vi "Main.vi"() -> ()   [LabVIEW 2019]
doc: "Simple string based state machine."
uses:
  <vilib>/Utility/error.llb/Error Cluster From Error Code.vi
  <vilib>/ErrorRing/Error Ring.xnode
  Support VIs/Communication/Queues/MHL/MHL.lvlib
  Support VIs/Modules/Deep Thought/Deep Thought.lvlib
  Support VIs/Communication/Notifiers/Sequencer/Sequencer Handshake.lvlib
panel:
  out "Deep Thought":string
  in  "Ultimate Question":bool
  in  "Ultimate Answer":bool
  in  "Stop":bool
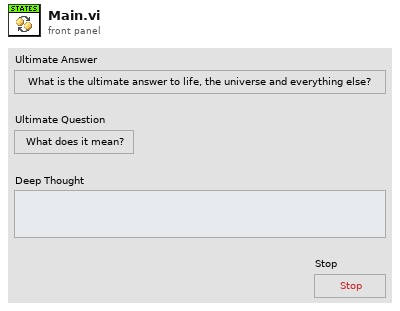
[diagram p1: front panel]
types:
  T1 = typedef "Events.ctl" = cluster{"Stop":refnum<user-event>}
  T2 = enum16{"Create Event", "Generate Event", "Destroy Event"}
  T3 = enum16{"Obtain", "Enqueue", "Get Queue", "Flush", "Release"}
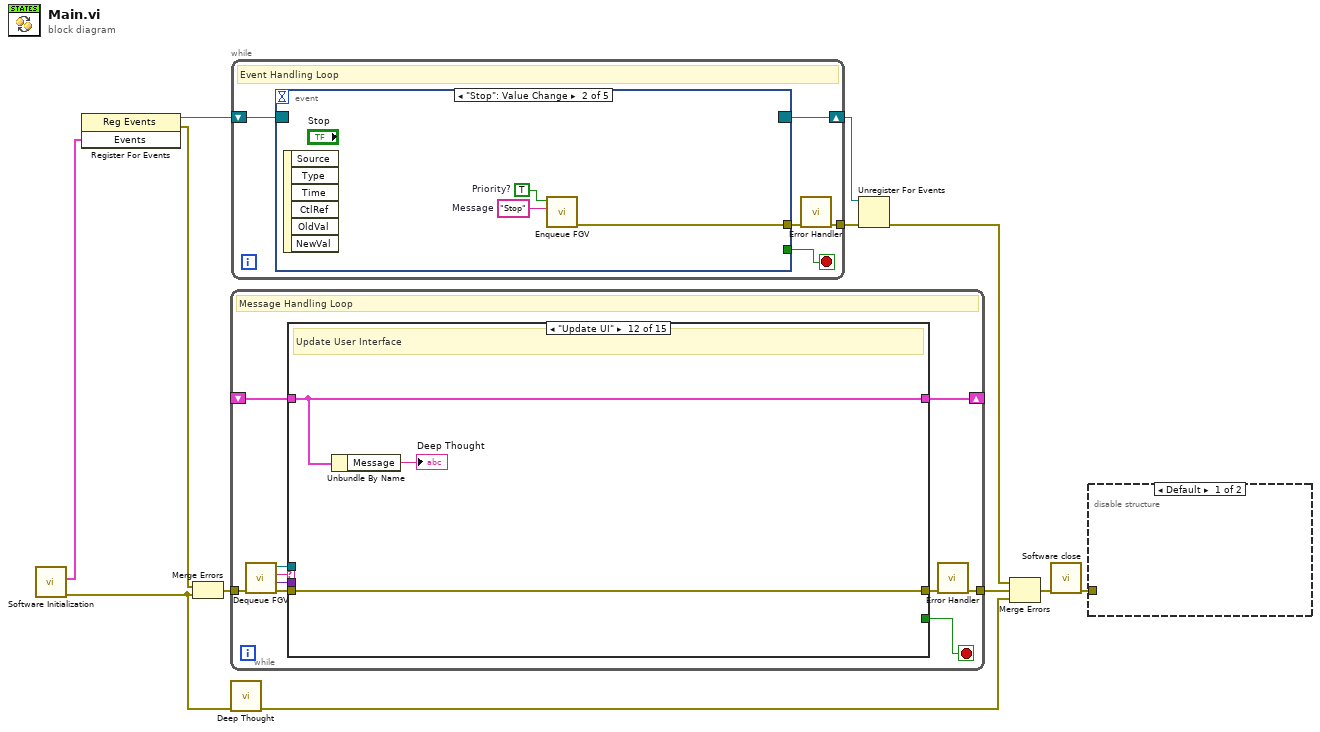
[diagram p0: block diagram]
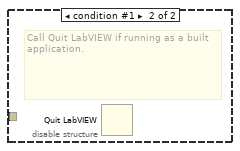
[diagram p2: hidden frame]
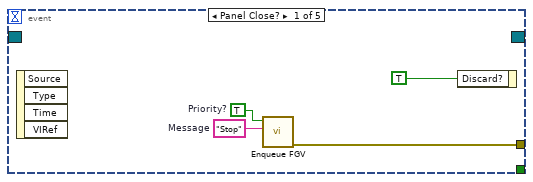
[diagram p3: hidden frame]
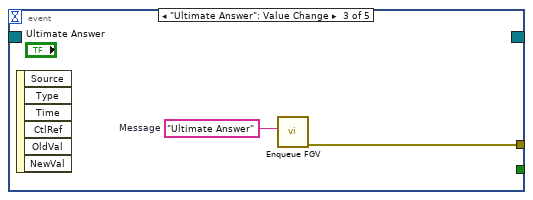
[diagram p4: hidden frame]
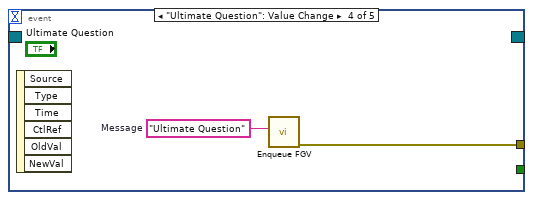
[diagram p5: hidden frame]
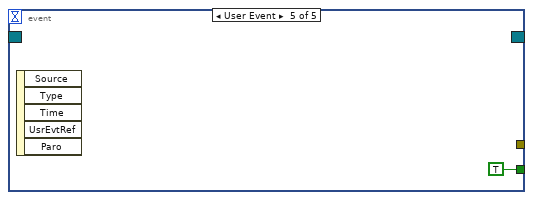
[diagram p6: hidden frame]
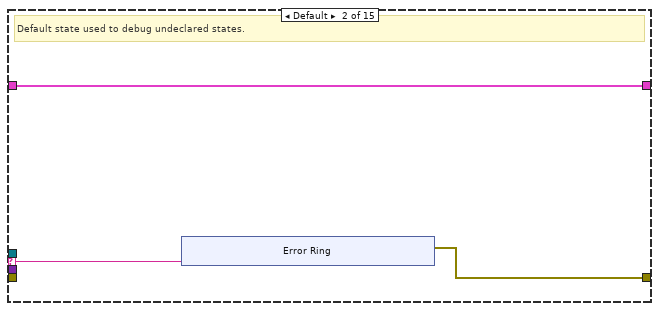
[diagram p8: hidden frame]
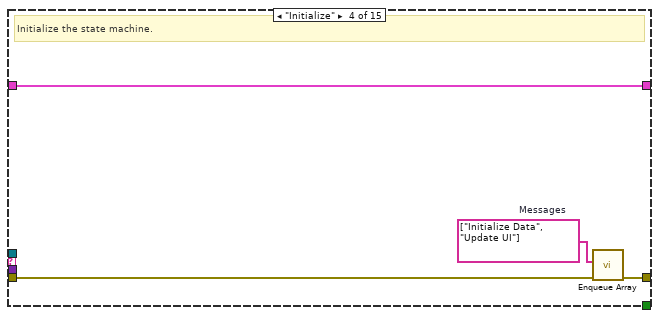
[diagram p10: hidden frame]
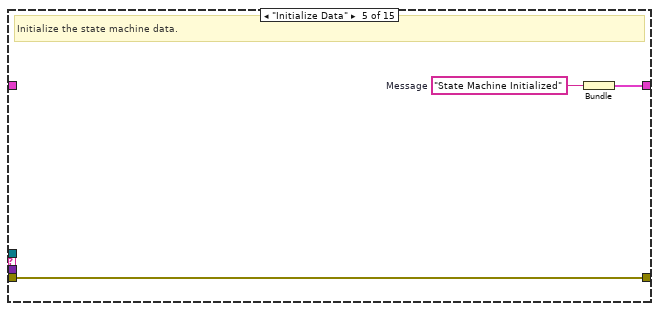
[diagram p11: hidden frame]
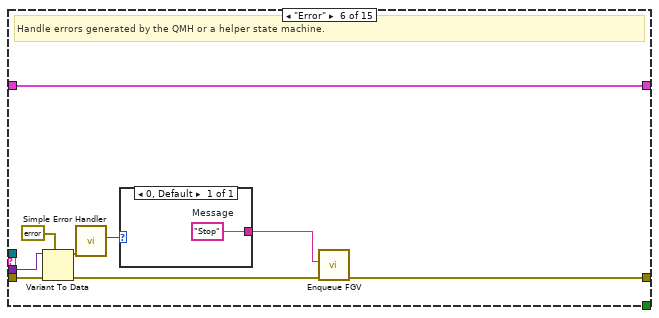
[diagram p12: hidden frame]
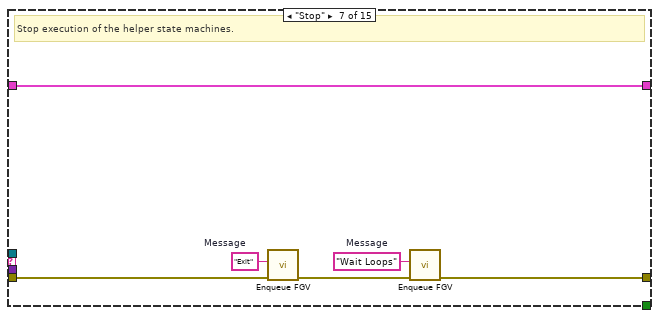
[diagram p13: hidden frame]
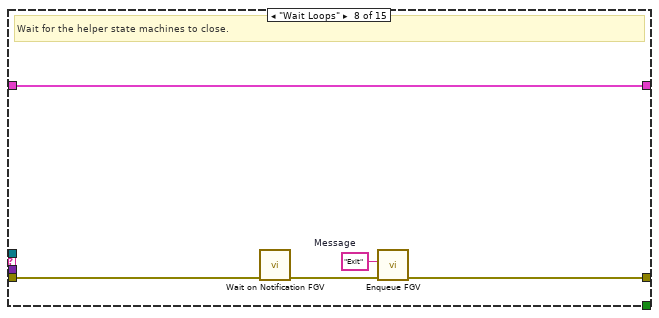
[diagram p14: hidden frame]
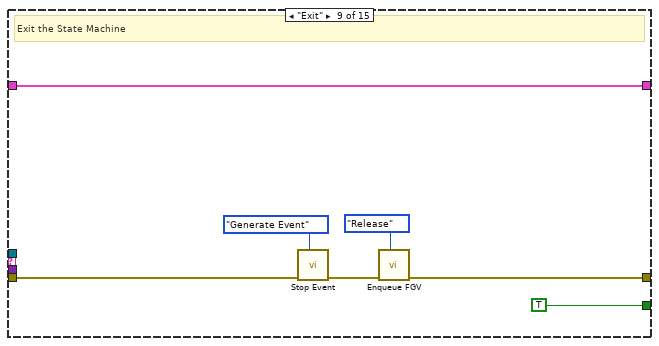
[diagram p15: hidden frame]
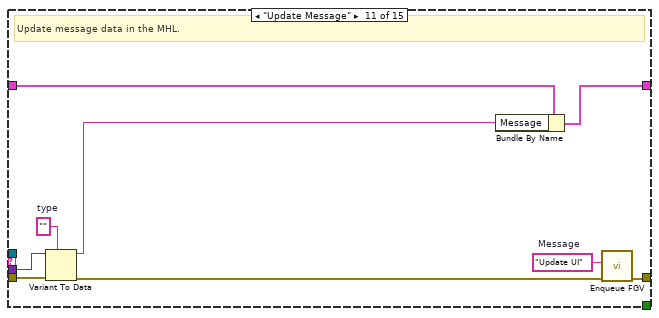
[diagram p17: hidden frame]
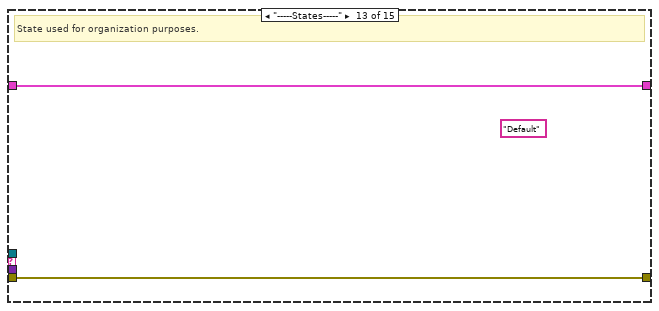
[diagram p18: hidden frame]
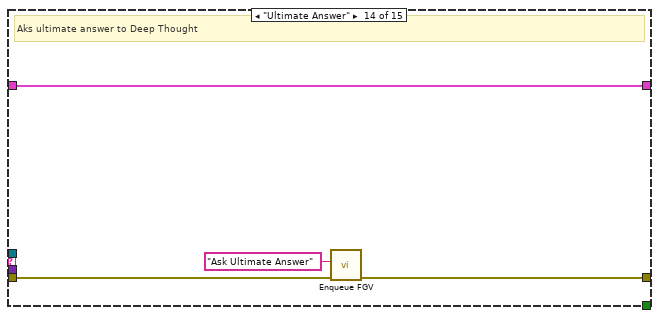
[diagram p19: hidden frame]
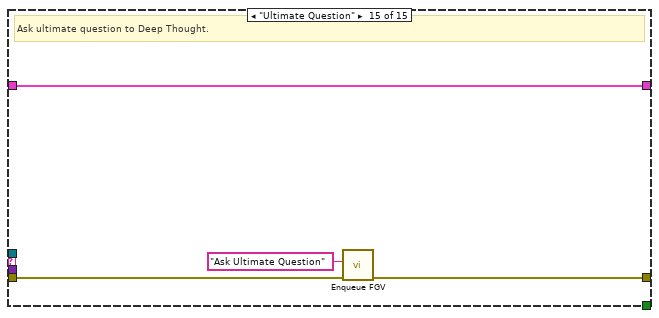
[diagram p20: hidden frame]
diagram:
  n1 = call "Software Initialization.vi"() -> ("error out"=w2:errorcluster, "Events"=w10:T1)  [unwired: 10 in]
  n2 = register-events(w10) -> (reference out=w11:refnum<event-registration>, error out=w8:errorcluster)  [unwired: 2 in]
  n3 = Merge Errors(w8, w2) -> (w9:errorcluster)
  n4 = while {
    shift-right: [w21] -> _
    shift-left: _ -> [w22]
    tunnel: w9 -> [w20]
    tunnel: [w18] -> w5
    stop <- w13 stop-if-true
    # "Message Handling Loop"
    n5 = call "Dequeue FGV.vi"("error in"=w20) -> ("error out"=w19:errorcluster, "Message Data"=w15:variant, "Message"=w16:string, "queue out"=w14:refnum<queue>)  [unwired: 7 in]
    n6 = case shown="\"Update UI\"" w16 {
      selector: w16 -> [_ w26 _ _ _ _ _ _ _ _ _ _ _ _ _]
      tunnel: w19 -> [w24 _ w36 w39 w41 w51 w56 w63 w66 w73 w80 w83 w87 w91 w95]
      tunnel: [w24 w25 w36 w40 w41 w46 w58 w61 w69 w73 w76 w83 w87 w90 w94] -> w17
      tunnel: [_ _ _ _ _ _ _ _ TRUE _ _ _ _ _ _] -> w13
      tunnel: w22 -> [w23 w27 w35 w37 _ w52 w59 w64 w70 w72 w82 w85 w86 w88 w92]
      tunnel: [w23 w27 w35 w37 w42 w52 w59 w64 w70 w72 w81 w85 w86 w88 w92] -> w21
      tunnel: w15 -> [_ _ _ _ _ w50 _ _ _ _ w79 _ _ _ _]
      tunnel: w14 -> [_ _ _ _ _ _ _ _ _ _ _ _ _ _ _]
      frame "-----Debug-----" {
        # "State used for organization purposes."
      }
      frame Default {
        # "Default state used to debug undeclared states."
        n7 = xnode "Error Ring"("parameter 0"=w26) -> ("error out"=w25:errorcluster)
      }
      frame "-----Core-----" {
        # "State used for organization purposes."
      }
      frame "Initialize" {
        w38 = string[] ["Initialize Data", "Update UI"]  # Messages
        # "Initialize the state machine."
        n8 = call "Enqueue Array.vi"("error in"=w39, "Messages"=w38) -> ("error out"=w40:errorcluster)  [unwired: 9 in]
      }
      frame "Initialize Data" {
        w43 = "State Machine Initialized"  # Message
        # "Initialize the state machine data."
        n9 = Bundle("Message"=w43) -> (w42:cluster{"Message":string})  [unwired: 1 in]
      }
      frame "Error" {
        # "Handle errors generated by the QMH or a helper state machine."
        n10 = Variant To Data(error in=w51, type=errorcluster {"status"=FALSE, "code"=0, "source"=""} ("error constant"), Variant=w50) -> (data=w48:errorcluster, error out=w47:errorcluster)
        n11 = call <vilib>:"Simple Error Handler.vi"("error in (no error)"=w48) -> ("code out"=w45:i32)  [unwired: 4 in, 4 out]
        n12 = case shown="0, Default" w45 {
          tunnel: [w53] -> w44
          frame 0, Default {
            w53 = "Stop"  # Message
          }
        }
        n13 = call "Enqueue FGV.vi"("error in"=w47, "Message"=w44) -> ("error out"=w46:errorcluster)  [unwired: 8 in, 1 out]
      }
      frame "Stop" {
        w54 = "Wait Loops"  # Message
        w55 = "Exit"  # Message
        # "Stop execution of the helper state machines."
        n14 = call "Enqueue FGV.vi"("error in"=w56, "Message"=w55) -> ("error out"=w57:errorcluster)  [unwired: 8 in, 1 out]
        n15 = call "Enqueue FGV.vi"("error in"=w57, "Message"=w54) -> ("error out"=w58:errorcluster)  [unwired: 8 in, 1 out]
      }
      frame "Wait Loops" {
        w60 = "Exit"  # Message
        # "Wait for the helper state machines to close."
        n16 = call "Wait on Notification FGV.vi"("error in"=w63) -> ("error out"=w62:errorcluster)  [unwired: 8 in, 2 out]
        n17 = call "Enqueue FGV.vi"("error in"=w62, "Message"=w60) -> ("error out"=w61:errorcluster)  [unwired: 8 in, 1 out]
      }
      frame "Exit" {
        # "Exit the State Machine"
        n18 = call "Stop Event.vi"("Actions"=T2."Generate Event", "error in"=w66) -> ("error out"=w65:errorcluster)  [unwired: 8 in, 1 out]
        n19 = call "Enqueue FGV.vi"("Actions"=T3."Release", "error in"=w65) -> ("error out"=w69:errorcluster)  [unwired: 8 in, 1 out]
      }
      frame "-----User Interface-----" {
        # "State used for organization purposes."
      }
      frame "Update Message" {
        w74 = "Update UI"  # Message
        w78 = ""  # type
        # "Update message data in the MHL."
        n20 = Variant To Data(error in=w80, type=w78, Variant=w79) -> (data=w77:string, error out=w75:errorcluster)
        n21 = Bundle By Name(cluster=w82, "Message"=w77) -> (w81:cluster{"Message":string})
        n22 = call "Enqueue FGV.vi"("error in"=w75, "Message"=w74) -> ("error out"=w76:errorcluster)  [unwired: 8 in, 1 out]
      }
      frame "Update UI" {
        # "Update User Interface"
        n23 = Unbundle By Name(w85) -> ("Message"=→"Deep Thought":string)
      }
      frame "-----States-----" {
        (unwired) "Default" ("State")
        # "State used for organization purposes."
      }
      frame "Ultimate Answer" {
        # "Aks ultimate answer to Deep Thought"
        n24 = call "Enqueue FGV.vi"("error in"=w91, "Message"="Ask Ultimate Answer") -> ("error out"=w90:errorcluster)  [unwired: 8 in, 1 out]
      }
      frame "Ultimate Question" {
        # "Ask ultimate question to Deep Thought."
        n25 = call "Enqueue FGV.vi"("error in"=w95, "Message"="Ask Ultimate Question") -> ("error out"=w94:errorcluster)  [unwired: 8 in, 1 out]
      }
    }
    n26 = call "Error Handler.vi"("error in"=w17) -> ("dup error in"=w18:errorcluster)  [unwired: 9 in, 1 out]
  }
  n27 = call "Deep Thought.vi"("Error In"=w2) -> ("Error Out"=w1:errorcluster)  [unwired: 10 in]
  n28 = while {
    shift-right: [w97] -> w6
    shift-left: w11 -> [w100]
    tunnel: [w98] -> w7
    stop <- w96 stop-if-true
    # "Event Handling Loop"
    n29 = event shown="[1] \"Stop\": Value Change" {
      selector: w100 -> [_ _ _ _ _]
      dyn-events: [_ _ _ _ _] -> w97
      timeout: _ -> [_ _ _ _ _]
      tunnel: [w103 w105 w108 w110 _] -> w99
      tunnel: [_ _ _ _ TRUE] -> w96
      event Panel Close? {
        w101 = "Stop"  # Message
        w102 = TRUE  # Priority?
        # "Panel Close event."
        n30 = event-data() -> ()  [unwired: 1 in, 4 out]
        n31 = call "Enqueue FGV.vi"("Message"=w101, "Priority?"=w102) -> ("error out"=w103:errorcluster)  [unwired: 8 in, 1 out]
        n32 = event-data("Discard?"=TRUE) -> ()  [unwired: 1 in, 1 out]
      }
      event "Stop": Value Change {
        w106 = "Stop"  # Message
        w107 = TRUE  # Priority?
        # "Stop button value change event."
        n33 = event-data() -> ()  [unwired: 1 in, 6 out]
        n34 = call "Enqueue FGV.vi"("Message"=w106, "Priority?"=w107) -> ("error out"=w105:errorcluster)  [unwired: 8 in, 1 out]
      }
      event "Ultimate Answer": Value Change {
        w109 = "Ultimate Answer"  # Message
        # "Ultimate Answer button value change event."
        n35 = event-data() -> ()  [unwired: 1 in, 6 out]
        n36 = call "Enqueue FGV.vi"("Message"=w109) -> ("error out"=w108:errorcluster)  [unwired: 9 in, 1 out]
      }
      event "Ultimate Question": Value Change {
        w111 = "Ultimate Question"  # Message
        # "Ultimate Question button value change event."
        n37 = event-data() -> ()  [unwired: 1 in, 6 out]
        n38 = call "Enqueue FGV.vi"("Message"=w111) -> ("error out"=w110:errorcluster)  [unwired: 9 in, 1 out]
      }
      event User Event {
        n39 = event-data() -> ()  [unwired: 1 in, 5 out]
      }
    }
    n40 = call "Error Handler.vi"("error in"=w99) -> ("dup error in"=w98:errorcluster)  [unwired: 9 in, 1 out]
  }
  n41 = Unregister For Events(event registration refnum=w6, error in=w7) -> (error out=w4:errorcluster)
  n42 = Merge Errors(w4, w5, w1) -> (w3:errorcluster)
  n43 = call "Software close.vi"("error in"=w3) -> ("error out"=w12:errorcluster)  [unwired: 10 in]
  n44 = disable-structure shown="Default" {
    disable-tunnel: w12 -> [_ _]
    frame condition #0 (active) {
    }
    frame condition #1 {
      # "Call Quit LabVIEW if running as a built application."
      n45 = Quit LabVIEW() -> ()  [unwired: 1 in]
    }
  }
